vi "Initialize.vi"(7 "ChannelName":string="Setpoint.ch%d.SP", 8 "error in":errorcluster, 9 "Number of Channels":u32=1, 10 "Instance Name":string, 11 "Parameter Set in":refnum<class "Parameter Set.lvclass">) -> (0 "error out":errorcluster, 2 "Channel":T1[](array[typedef]), 3 "Parameter Set out":refnum<class "Parameter Set.lvclass">)   [LabVIEW 2023, in "Parameter Set.lvclass"]
uses:
  Parameter Set.lvclass
  Utilities/Channel.ctl
  Parameter Set.lvclass/Parameter Set.ctl
  <vilib>/ADAS Replay HIL/Channels/Tag Wrapper/Polymorphic/Open Producer Tag (I32).vi
  <vilib>/ADAS Replay HIL/Channels/Tag Wrapper/Polymorphic/Set Default Value (I32).vi
  <vilib>/ADAS Replay HIL/Channels/Tag Wrapper/Polymorphic/Open Consumer Tag (I32).vi
  <vilib>/ADAS Replay HIL/Channels/Tag Wrapper/Polymorphic/Open Producer Tag (I32).vi/45cd6eaa-a1ce-41a4-8aba-62a49d103d7e.vi
  <vilib>/ADAS Replay HIL/Channels/Tag Wrapper/Polymorphic/Set Default Value (I32).vi/228e99de-6fcf-414d-86fc-dc277c7b351f.vi
  <vilib>/ADAS Replay HIL/Channels/Tag Wrapper/Polymorphic/Open Consumer Tag (I32).vi/bacb721e-673a-491a-accd-959f2e1f334e.vi
  <vilib>/ADAS Replay HIL/Channels/Tag Wrapper/Polymorphic/Open Producer Tag (I32).vi/45cd6eaa-a1ce-41a4-8aba-62a49d103d7e.vi/c28b0ead-42ad-4072-80a2-aca7f2bd7ce3.vi
  <vilib>/ADAS Replay HIL/Channels/Tag Wrapper/Polymorphic/Set Default Value (I32).vi/228e99de-6fcf-414d-86fc-dc277c7b351f.vi/4bc1c15b-36ab-481f-b8dd-c64075ce723a.vi
  <vilib>/ADAS Replay HIL/Channels/Tag Wrapper/Polymorphic/Open Consumer Tag (I32).vi/bacb721e-673a-491a-accd-959f2e1f334e.vi/c28b0ead-42ad-4072-80a2-aca7f2bd7ce3.vi
  <vilib>/ADAS Replay HIL/AdasHilServices/AdasHilServices Fill In Error Info Ex.vi
  adas-replay-hil-internal/source/Channels/Tag Wrapper/Tag Wrapper.lvlib
  Utilities/Utilities.lvlib
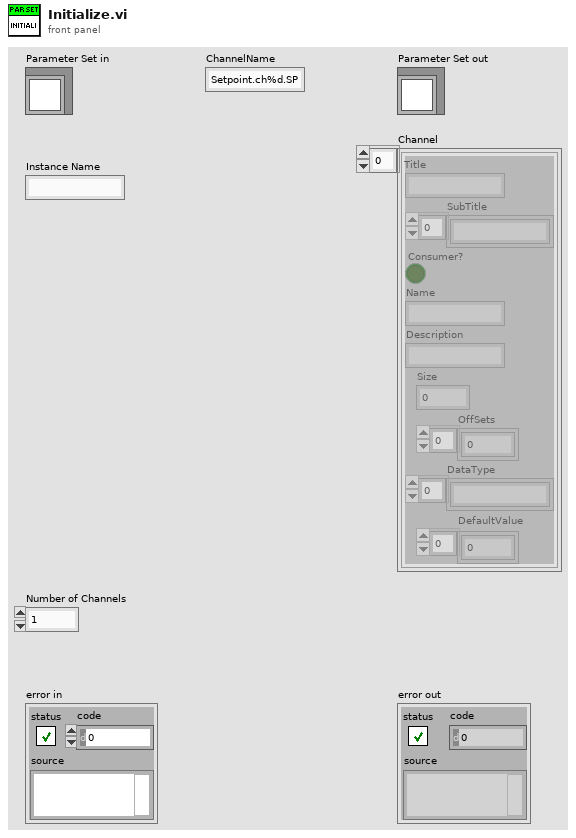
[diagram p1: front panel]
types:
  T1 = typedef "Utilities.lvlib/Channel.ctl" = cluster{"Title":string, "SubTitle":string[], "Consumer?":bool, "Name":string, "Description":string, "Size":i32, "OffSets":i32[], "DataType":string[], "DefaultValue":dbl[]}
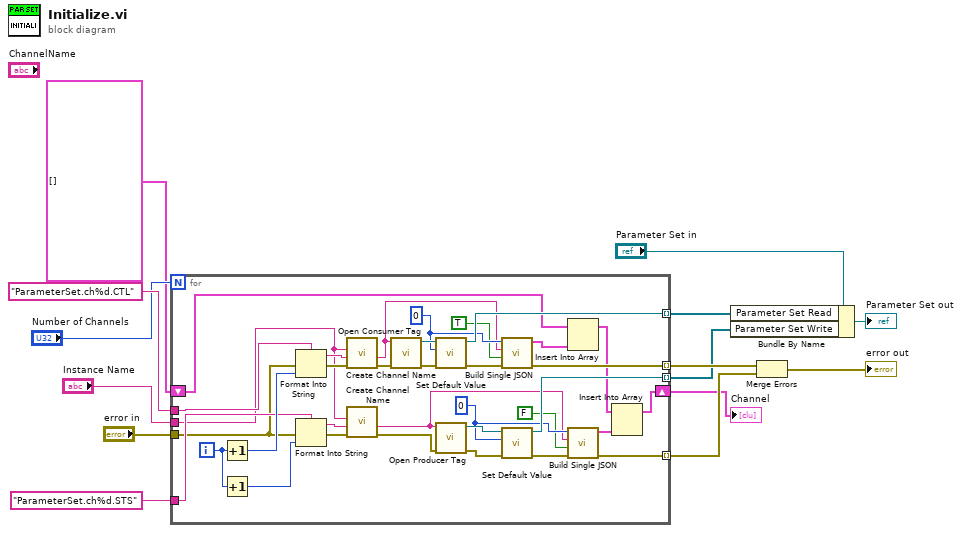
[diagram p0: block diagram]
diagram:
  n1 = for {
    N: "Number of Channels" -> [_]
    tunnel: "ParameterSet.ch%d.CTL" ("ChannelName") -> [w47]
    tunnel: "error in" -> [w31]
    tunnel: [w21] -> w12 mode=indexing
    tunnel: [w28] -> w13 mode=indexing
    tunnel: "ParameterSet.ch%d.STS" ("ChannelName") -> [w38]
    tunnel: [w36] -> w14 mode=indexing
    tunnel: [w35] -> w11 mode=indexing
    tunnel: "Instance Name" -> [w30]
    shift-right: [w16] -> w1
    shift-left: T1[] [] -> [w15]
    i -> [w39]
    w26 = 0 ("Default Value")
    w27 = 0 ("Default Value")
    n2 = Increment(x=w39) -> (x+1=w48:i32)
    n3 = Increment(x=w39) -> (x+1=w40:i32)
    n4 = Format Into String(format string=w47, error in=w31, w48) -> (resulting string=w46:string, error out=w33:errorcluster)  [unwired: 1 in]
    n5 = Format Into String(format string=w38, error in=w31, w40) -> (resulting string=w37:string, error out=w32:errorcluster)  [unwired: 1 in]
    n6 = call "Create Channel Name.vi"("error in"=w33, "Channel Name"=w46, "Plugin Name"=w30) -> ("error out"=w34:errorcluster, "Data Channel Name"=w24:string)  [unwired: 7 in]
    n7 = call "Create Channel Name.vi"("error in"=w32, "Channel Name"=w37, "Plugin Name"=w30) -> ("error out"=w42:errorcluster, "Data Channel Name"=w25:string)  [unwired: 7 in]
    n8 = call-poly <vilib>:"Open Consumer Tag.vi"("error in"=w34, "Channel Name"=w24) -> ("error out"=w44:errorcluster, "ADAS HIL Channel"=w45:refnum<k21>)  [unwired: 8 in]
    n9 = call-poly <vilib>:"Set Default Value.vi"("error in"=w44, "Default Value"=w27, "ADAS HIL Channel in"=w45) -> ("error out"=w22:errorcluster, "ADAS HIL Channel out"=w36:refnum<k21>)  [unwired: 7 in]
    n10 = call-poly <vilib>:"Open Producer Tag.vi"("error in"=w42, "Channel Name"=w25) -> ("error out"=w41:errorcluster, "ADAS HIL Channel"=w43:refnum<k21>)  [unwired: 8 in]
    n11 = call "Build Single JSON.vi"("error in"=w22, "Consumer?"=TRUE, "ChannelName"=w24, "Single"=w27) -> ("error out"=w21:errorcluster, "Channel"=w19:T1)  [unwired: 6 in]
    n12 = call-poly <vilib>:"Set Default Value.vi"("error in"=w41, "Default Value"=w26, "ADAS HIL Channel in"=w43) -> ("error out"=w29:errorcluster, "ADAS HIL Channel out"=w35:refnum<k21>)  [unwired: 7 in]
    n13 = Insert Into Array(array=w15, new element=w19) -> (w17:T1[])  [unwired: 1 in]
    n14 = call "Build Single JSON.vi"("error in"=w29, "Consumer?"=FALSE, "ChannelName"=w25, "Single"=w26) -> ("error out"=w28:errorcluster, "Channel"=w18:T1)  [unwired: 6 in]
    n15 = Insert Into Array(array=w17, new element=w18) -> (w16:T1[])  [unwired: 1 in]
  }
  "Channel" <- w1
  n16 = Bundle By Name(cluster="Parameter Set in", "Parameter Set Read"=w14, "Parameter Set Write"=w11) -> (→"Parameter Set out":refnum<class "Parameter Set.lvclass">)
  n17 = Merge Errors(w12, w13) -> (→"error out":errorcluster)
